vi "write_attributes.vi"(8 "error in (no error)":errorcluster, 10 "attributes":T1, 11 "StackingClassifier in":refnum<class "StackingClassifier.lvclass">) -> (0 "error out":errorcluster, 3 "StackingClassifier out":refnum<class "StackingClassifier.lvclass">)   [LabVIEW 2020, in "StackingClassifier.lvclass"]
uses:
  StackingClassifier.lvclass
  Controls/stacking_classifier_attributes.ctl
  StackingClassifier.lvclass/StackingClassifier.ctl
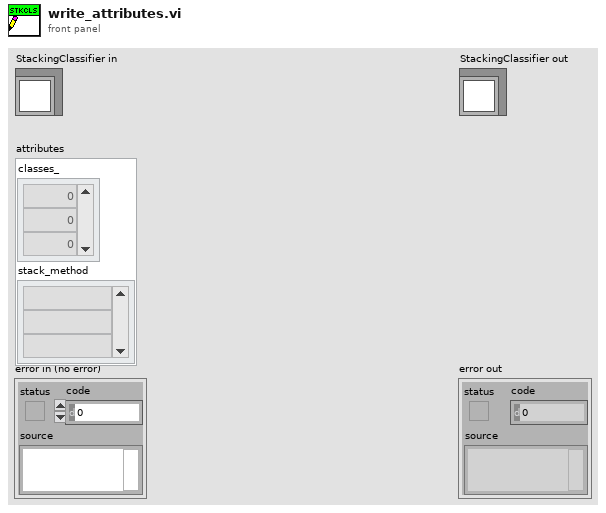
[diagram p1: front panel]
types:
  T1 = typedef "stacking_classifier_attributes.ctl" = cluster{"classes_":dbl[], "stack_method":string[]}
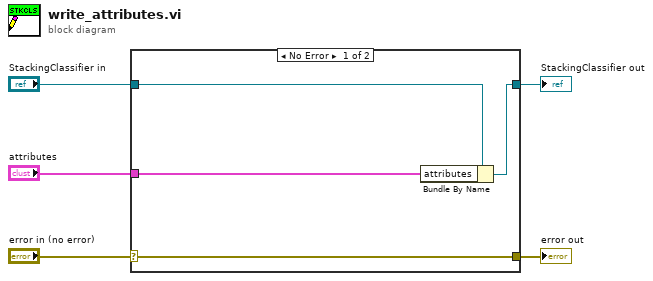
[diagram p0: block diagram]
diagram:
  n1 = case shown="No Error" "error in (no error)" {
    selector: "error in (no error)" -> [w9 w10]
    tunnel: [w9 w10] -> w4
    tunnel: [w7 w11] -> w2
    tunnel: "StackingClassifier in" -> [w8 w11]
    tunnel: "attributes" -> [w6 _]
    frame No Error {
      n2 = Bundle By Name(cluster=w8, "attributes"=w6) -> (w7:refnum<class "StackingClassifier.lvclass">)
    }
    frame Error {
    }
  }
  "error out" <- w4
  "StackingClassifier out" <- w2
